vi "P4CMD Get Project Name.vi"(2 "config data in":string) -> (7 "project name":string)   [LabVIEW 2017, in "NI_SCC_P4CMD.lvlib"]
uses:
  <vilib>/SourceControl/Providers/P4CMD/NI_SCC_P4CMD.lvlib
  <vilib>/SourceControl/support/SCCSup ConfigData Conv.ctl
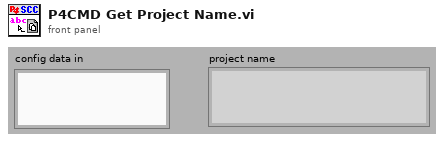
[diagram p1: front panel]
types:
  T1 = typedef "SCCSup ConfigData Conv.ctl" = enum16{"from config data", "to config data"}
  T2 = typedef "NI_SCC_P4CMD.lvlib/P4CMD SCC Config Info.ctl" = cluster{"GBL lock on checkout?":bool, "GBL suppress dlgs?":bool, "port":string, "client":string, "user":string, "password":string}
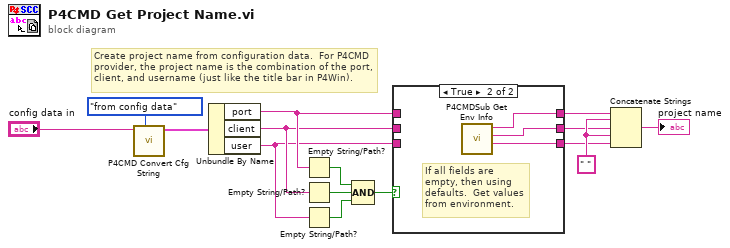
[diagram p0: block diagram]
diagram:
  w11 = " "
  # "Create project name from configuration data.  For P4CMD provider, the project name is the combination of the port, client, and username (just like the title bar in P4Win)."
  n1 = call <vilib>:"P4CMD Convert Cfg String.vi"("conversion action"=SCCSup_ConfigData_Conv."from config data", "config data in"="config data in") -> ("configuration details out"=w12:T2)  [unwired: 7 in, 2 out]
  n2 = Unbundle By Name(w12) -> ("port"=w6:string, "client"=w5:string, "user"=w4:string)
  n3 = Empty String/Path?(string/path=w6) -> (empty?=w10:bool)
  n4 = Empty String/Path?(string/path=w5) -> (empty?=w9:bool)
  n5 = Empty String/Path?(string/path=w4) -> (empty?=w8:bool)
  n6 = Compound Arithmetic op=AND(w10, w9, w8) -> (w7:bool)
  n7 = case shown="True" w7 {
    tunnel: w6 -> [w18 _]
    tunnel: w5 -> [w17 _]
    tunnel: w4 -> [w16 _]
    tunnel: [w18 w21] -> w3
    tunnel: [w17 w20] -> w2
    tunnel: [w16 w19] -> w1
    frame False {
    }
    frame True {
      # "If all fields are empty, then using defaults.  Get values from environment."
      n8 = call <vilib>:"P4CMDSub Get Env Info.vi"() -> ("user"=w19:string, "client"=w20:string, "port"=w21:string)  [unwired: 8 in, 1 out]
    }
  }
  n9 = Concatenate Strings(w3, w11, w2, w11, w1) -> (→"project name":string)
